vi "Read.vi"(8 "error in (no error)":errorcluster, 10 "Number Of Bytes":i32, 11 "VISA resource name":refnum<visa-resource-name>) -> (0 "error out":errorcluster, 1 "String":string, 2 "Returned Bytes":i32, 3 "VISA resource name out":refnum<visa-resource-name>)   [LabVIEW 2022 SP3, in "Agilent ENA Series.lvlib"]
doc: "Reads a lot of bytes from instrument and prevent to timeout error occurred."
uses:
  <instrlib>/Agilent Ena Series/Agilent ENA Series.lvlib
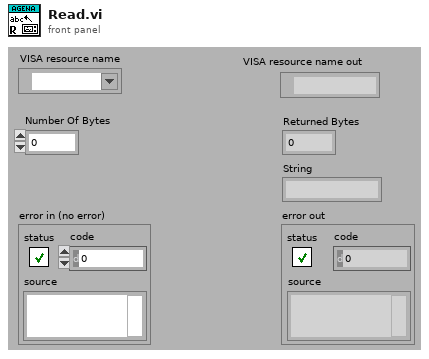
[diagram p1: front panel]
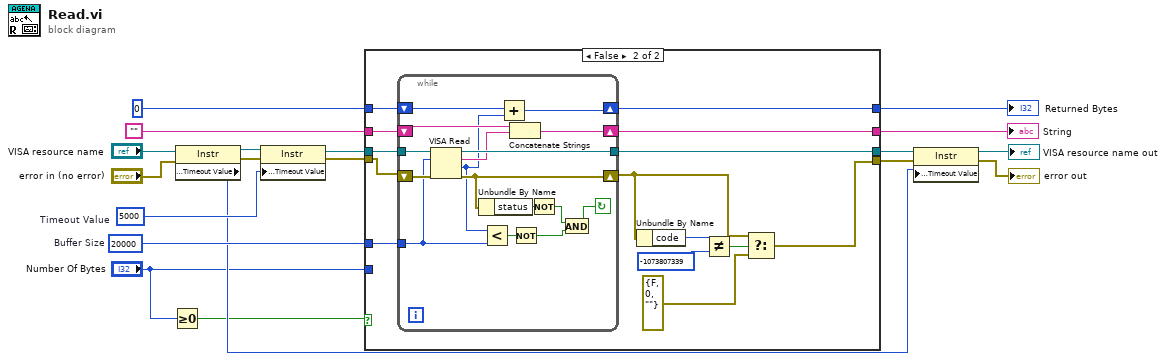
[diagram p0: block diagram]
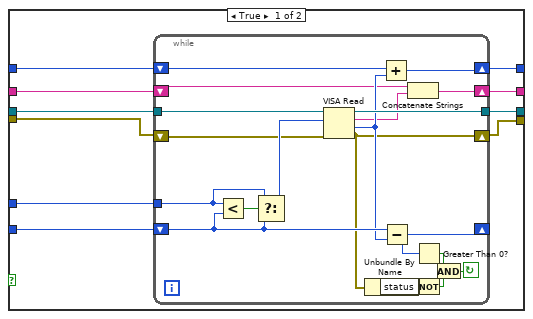
[diagram p2: hidden frame]
diagram:
  w10 = u32 5000  # Timeout Value
  w17 = u32 20000  # Buffer Size
  n1 = Greater Or Equal To 0?(x="Number Of Bytes") -> (x >= 0?=w2:bool)
  n2 = property class="Instr"(reference="VISA resource name", error in="error in (no error)") -> (reference out=w12:refnum<visa-resource-name>, error out=w11:errorcluster, "General Settings:Timeout Value"=w4:u32)
  n3 = property class="Instr"(reference=w12, error in=w11, "General Settings:Timeout Value"=w10) -> (reference out=w8:refnum<visa-resource-name>, error out=w9:errorcluster)
  n4 = case shown="False" w2 {
    tunnel: "" -> [w29 w62]
    tunnel: [w28 w61] -> w18
    tunnel: w17 -> [w27 w60]
    tunnel: "Number Of Bytes" -> [w26 _]
    tunnel: u32 0 ("byte count (0)") -> [w25 w59]
    tunnel: [w24 w58] -> w15
    tunnel: w9 -> [w23 w57]
    tunnel: w8 -> [w22 w56]
    tunnel: [w21 w55] -> w7
    tunnel: [w20 w49] -> w6
    frame True {
      n5 = while {
        shift-left: w29 -> [w33]
        shift-right: [w34] -> w24
        tunnel: w27 -> [w42]
        shift-left: w25 -> [w40]
        shift-right: [w39] -> w28
        shift-left: w26 -> [w44]
        shift-right: [w43] -> _
        shift-left: w23 -> [w30]
        shift-right: [w31] -> w20
        tunnel: [w47] -> w21
        tunnel: w22 -> [w48]
        stop <- w35 continue-if-true
        n6 = Less?(x=w42, y=w44) -> (x < y?=w46:bool)
        n7 = Select(t=w42, s=w46, f=w44) -> (s? t:f=w45:u32)
        n8 = VISA Read(VISA resource name=w48, byte count=w45, error in (no error)=w30) -> (VISA resource name out=w47:refnum<visa-resource-name>, read buffer=w32:string, return count=w41:u32, error out=w31:errorcluster)
        n9 = Unbundle By Name(w31) -> ("status"=w37:bool)
        n10 = Add(x=w40, y=w41) -> (x+y=w39:u32)
        n11 = Subtract(x=w44, y=w41) -> (x-y=w43:u32)
        n12 = Concatenate Strings(w33, w32) -> (w34:string)
        n13 = Greater Than 0?(x=w43) -> (x > 0?=w38:bool)
        n14 = Not(x=w37) -> (.not. x?=w36:bool)
        n15 = And(x=w38, y=w36) -> (x .and. y?=w35:bool)
      }
    }
    frame False {
      n16 = while {
        shift-left: w62 -> [w72]
        shift-right: [w73] -> w58
        tunnel: w60 -> [w63]
        shift-left: w59 -> [w76]
        shift-right: [w75] -> w61
        shift-left: w57 -> [w69]
        shift-right: [w70] -> w51
        tunnel: [w77] -> w55
        tunnel: w56 -> [w78]
        stop <- w65 continue-if-true
        n17 = VISA Read(VISA resource name=w78, byte count=w63, error in (no error)=w69) -> (VISA resource name out=w77:refnum<visa-resource-name>, read buffer=w71:string, return count=w64:u32, error out=w70:errorcluster)
        n18 = Unbundle By Name(w70) -> ("status"=w74:bool)
        n19 = Less?(x=w64, y=w63) -> (x < y?=w68:bool)
        n20 = Add(x=w76, y=w64) -> (x+y=w75:u32)
        n21 = Concatenate Strings(w72, w71) -> (w73:string)
        n22 = Not(x=w68) -> (.not. x?=w67:bool)
        n23 = Not(x=w74) -> (.not. x?=w66:bool)
        n24 = And(x=w66, y=w67) -> (x .and. y?=w65:bool)
      }
      n25 = Unbundle By Name(w51) -> ("code"=w54:i32)
      n26 = Not Equal?(x=w54, y=-1073807339) -> (x != y?=w52:bool)
      n27 = Select(t=w51, s=w52, f=errorcluster {"status"=FALSE, "code"=0, "source"=""}) -> (s? t:f=w49:errorcluster)
    }
  }
  "Returned Bytes" <- w18
  "String" <- w15
  n28 = property class="Instr"(reference=w7, error in=w6, "General Settings:Timeout Value"=w4) -> (reference out=→"VISA resource name out":refnum<visa-resource-name>, error out=→"error out":errorcluster)
